vi "Get Signal Channels.vi"(9 "Signal Index":i32, 10 "QObject Refnum":u64, 11 "Signal Map":variant) -> (2 "Signal Channels":variant[](array[variant]), 3 "Dup. Signal Map":variant)   [LabVIEW 2013, in "Template.lvlib" / "LQCoreEngine.lvclass"]
uses:
  LQCoreEngine.lvclass
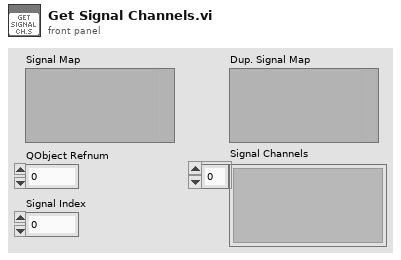
[diagram p1: front panel]
types:
  T1 = enum16{"big-endian, network order", "native, host order", "little-endian"}
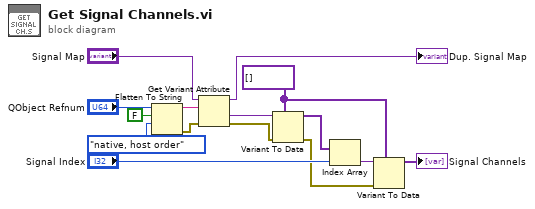
[diagram p0: block diagram]
diagram:
  w6 = variant[] []
  n1 = Flatten To String(anything="QObject Refnum", prepend array or string size? (T)=FALSE, byte order (0:big-endian, network order)=T1."native, host order") -> (data string=w11:string, error out=w4:errorcluster)  [unwired: 1 in, 1 out]
  n2 = Get Variant Attribute(Variant="Signal Map", name=w11, error in=w4) -> (duplicate Variant=→"Dup. Signal Map":variant, value=w10:variant, error out=w3:errorcluster)  [unwired: 1 in, 1 out]
  n3 = Variant To Data(error in=w3, type=w6, Variant=w10) -> (data=w9:variant[], error out=w5:errorcluster)
  n4 = Index Array(array=w9, index="Signal Index") -> (element=w7:variant)
  n5 = Variant To Data(error in=w5, type=w6, Variant=w7) -> (data=→"Signal Channels":variant[])  [unwired: 1 out]
